vi "Positioning Loop (SubVI).vi"   [LabVIEW 2015]
uses:
  Left Variables.vi
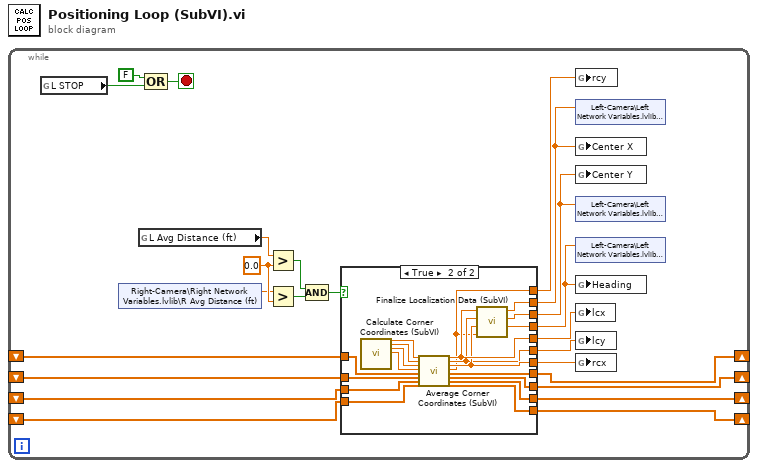
[diagram p0: block diagram]
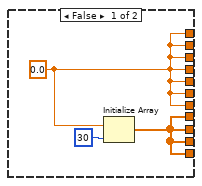
[diagram p2: hidden frame]
diagram:
  n1 = while {
    shift-right: [w15] -> _
    shift-left: _ -> [w11]
    shift-right: [w14] -> _
    shift-left: _ -> [w10]
    shift-right: [w13] -> _
    shift-left: _ -> [w9]
    shift-right: [w12] -> _
    shift-left: _ -> [w8]
    stop <- w23 stop-if-true
    w20 = 0.0 ("y")
    n2 = global read "Left Variables.vi" "L STOP"() -> (w21:bool)
    n3 = shared-variable "Right-Camera\\Right Network Variables.lvlib\\R Avg Distance (ft)"() -> (w17:dbl)  [unwired: 1 in, 1 out]
    n4 = global read "Left Variables.vi" "L Avg Distance (ft)"() -> (w18:dbl)
    n5 = Compound Arithmetic op=OR(FALSE, w21) -> (w23:bool)
    n6 = Greater?(x=w18, y=w20) -> (0:w19:bool)
    n7 = Greater?(x=w17, y=w20) -> (0:w16:bool)
    n8 = Compound Arithmetic op=AND(w19, w16) -> (w22:bool)
    n9 = case shown="True" w22 {
      tunnel: [w26 w43] -> w15
      tunnel: [w26 w42] -> w14
      tunnel: [w26 w41] -> w13
      tunnel: [w26 w40] -> w12
      tunnel: w11 -> [_ w46]
      tunnel: w10 -> [_ w45]
      tunnel: w9 -> [_ w44]
      tunnel: w8 -> [_ w35]
      tunnel: [w25 w39] -> w7
      tunnel: [w25 w37] -> w6
      tunnel: [w25 w38] -> w5
      tunnel: [w25 w36] -> w4
      tunnel: [w25 w34] -> w2
      tunnel: [w25 w33] -> w1
      tunnel: [w25 w32] -> w3
      frame False {
        w25 = 0.0 ("element")
        n10 = Initialize Array(w25, 30 ("dimension size")) -> (w26:dbl[])
      }
      frame True {
        n11 = call "Calculate Corner Coordinates (SubVI).vi"() -> ("lcx1"=w31:dbl, "lcy1"=w30:dbl, "rcx1"=w29:dbl, "rcy1"=w28:dbl)  [unwired: 20 in, 4 out]
        n12 = call "Average Corner Coordinates (SubVI).vi"("Raw lcx"=w31, "Raw lcy"=w30, "Raw rcx"=w29, "Raw rcy"=w28, "Input lcx Array"=w46, "Input lcy Array"=w45, "Input rcx Array"=w44, "Input rcy Array"=w35) -> ("Avg lcx"=w39:dbl, "Avg lcy"=w37:dbl, "Avg rcx"=w38:dbl, "Avg rcy"=w36:dbl, "Output lcx Array"=w43:dbl[], "Output lcy Array"=w42:dbl[], "Output rcx Array"=w41:dbl[], "Output rcy Array"=w40:dbl[])  [unwired: 12 in]
        n13 = call "Finalize Localization Data (SubVI).vi"("Avg rcy"=w36, "Avg rcx"=w38, "Avg lcy"=w37, "Avg lcx"=w39) -> ("Heading"=w32:dbl, "Center Y"=w33:dbl, "Center X"=w34:dbl)  [unwired: 5 in]
      }
    }
    n14 = global write "Left Variables.vi" "rcy"(w4) -> ()
    n15 = shared-variable "Left-Camera\\Left Network Variables.lvlib\\Center X"(w2) -> ()  [unwired: 1 in, 1 out]
    n16 = global write "Left Variables.vi" "Center X"(w2) -> ()
    n17 = global write "Left Variables.vi" "Center Y"(w1) -> ()
    n18 = shared-variable "Left-Camera\\Left Network Variables.lvlib\\Center Y"(w1) -> ()  [unwired: 1 in, 1 out]
    n19 = shared-variable "Left-Camera\\Left Network Variables.lvlib\\Heading"(w3) -> ()  [unwired: 1 in, 1 out]
    n20 = global write "Left Variables.vi" "Heading"(w3) -> ()
    n21 = global write "Left Variables.vi" "lcx"(w7) -> ()
    n22 = global write "Left Variables.vi" "lcy"(w6) -> ()
    n23 = global write "Left Variables.vi" "rcx"(w5) -> ()
  }
